vi "Periodic Tasks.vi"(8 "error in":errorcluster) -> ()   [LabVIEW 2017]
doc: "This VI runs in parallel to other tasks. It can contain as many user-defined periodic loops as you need. These can carry out PID or other sorts of timed response."
uses:
  <vilib>/Rock Robotics/WPI/Solenoid/WPI_SolenoidChannel.ctl
  Public/Documents/Cross The Road Electronics/Phoenix-LabVIEW/Motor Controller/Controls/CTRE_Phoenix_MotorControl_ControlMode.ctl
  <vilib>/Rock Robotics/WPI/Utilities/WPI_GetSetVariantRefNum.vi
  Robot Global Data.vi
  <vilib>/Rock Robotics/WPI/ThirdParty/Phoenix-LabVIEW/Motor Controller/Get/CTRE_Phoenix_MotorController_GetSelectedSensorData.vi
  <vilib>/Rock Robotics/Network Tables/NT Read String.vi
  <vilib>/Rock Robotics/WPI/Solenoid/WPI_SolenoidOpenSingle.vi
  <vilib>/Rock Robotics/WPI/Solenoid/WPI_SolenoidSetEnum.vi
  <vilib>/Rock Robotics/Network Tables/NT Read Number.vi
panel:
  out "Velocity (Raw Sensor Units per 100 ms)":i32(graph)
  in  "Min Turret":dbl
  in  "Max Turret":dbl
  in  "Min Arm":dbl
  in  "Max Arm":dbl
  in  "Min Pivot":dbl
  in  "Max Pivot":dbl
  in  "Pivot Magic?":bool=TRUE
  in  "Set Pivot Constants":bool
  in  "Pivot Constants":T1
  out "Arm Extension":i32
  out "Pivot Position":i32
  out "Turret Position":i32
  in  "Retract Solenoid Channel":T2
  out "Compressor Monitoring":bool
  out "Compressor Running":bool
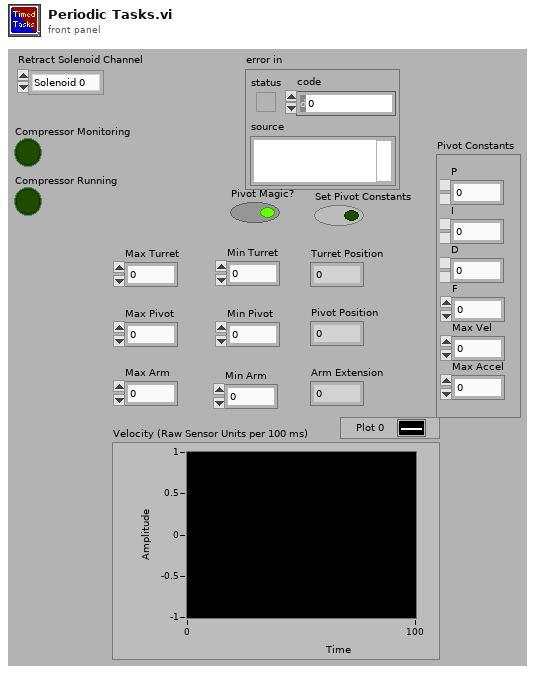
[diagram p1: front panel]
types:
  T1 = cluster{"P":dbl, "I":dbl, "D":dbl, "F":dbl, "Max Vel":dbl, "Max Accel":dbl}
  T2 = typedef "WPI_SolenoidChannel.ctl" = enum8{"Solenoid 0", "Solenoid 1", "Solenoid 2", "Solenoid 3", "Solenoid 4", "Solenoid 5", "Solenoid 6", "Solenoid 7", "Invalid"}
  T3 = typedef "WPI_CompressorDevRef.ctl" = cluster{"DevStatus":errorcluster, "Pneumatics Control Module":u8}
  T4 = typedef "WPI_SolenoidDevRef.ctl" = cluster{"DevStatus":errorcluster, "Pneumatics Control Module":u8, "Forward Solenoid Channel":T2, "Reverse Solenoid Channel":T2}
  T5 = typedef "WPI_MotorControlDeviceRef.ctl" = cluster{"DeviceStatus":errorcluster, "Type":T6, "PWM":cluster{"PWM Channel":T7, "DeadBand":T8}, "CAN":cluster{"Device Number":u8, "SetOutput VI Ref":variant, "GetOutput VI Ref":variant, "Enable VI Ref":variant, "Disable VI Ref":variant, "Data":variant}, "Invert":bool, "DIO PWM":cluster{"PWM \"Enable\" Channel":T7, "DIOChannel":T9, "PWM Rate":dbl}}
  T6 = typedef "WPI_MotorControlType.ctl" = enum16{"PWM", "CAN", "DIO PWM"}
  T7 = typedef "FPGA_DIOPWMChannel.ctl" = enum8{"PWM 0", "PWM 1", "PWM 2", "PWM 3", "PWM 4", "PWM 5", "PWM 6", "PWM 7", "PWM 8", "PWM 9", "PWM MXP 0", "PWM MXP 1", "PWM MXP 2", "PWM MXP 3", "PWM MXP 4", "PWM MXP 5", "PWM MXP 6", "PWM MXP 7", "PWM MXP 8", "PWM MXP 9", "Invalid"}
  T8 = typedef "WPI_PWMDeadband.ctl" = cluster{"Name":string, "maxPositivePwm":i32, "minPositivePwm":i32, "centerPwm":i32, "maxNegativePwm":i32, "minNegativePwm":i32, "angularRange":u16}
  T9 = typedef "FPGA_DIOChannel.ctl" = enum8{"DIO 0", "DIO 1", "DIO 2", "DIO 3", "DIO 4", "DIO 5", "DIO 6", "DIO 7", "DIO 8", "DIO 9", "DIO MXP 0", "DIO MXP 1", "DIO MXP 2", "DIO MXP 3", "DIO MXP 4", "DIO MXP 5", "DIO MXP 6", "DIO MXP 7", "DIO MXP 8", "DIO MXP 9", "DIO MXP 10", "DIO MXP 11", "DIO MXP 12", "DIO MXP 13", "DIO MXP 14", "DIO MXP 15", "SPI Port CS1", "SPI Port CS2", "SPI Port CS3", "SPI Port MISO", "SPI Port MOSI", "Invalid"}
  T10 = typedef "CTRE_Phoenix_MotorControl_ControlMode.ctl" = u16
  T11 = typedef "WPI_JoystickDevRef.ctl" = cluster{"Device":T12}
  T12 = typedef "WPI_JoystickDeviceEnum.ctl" = enum16{"USB 0", "USB 1", "USB 2", "USB 3", "USB 4", "USB 5"}
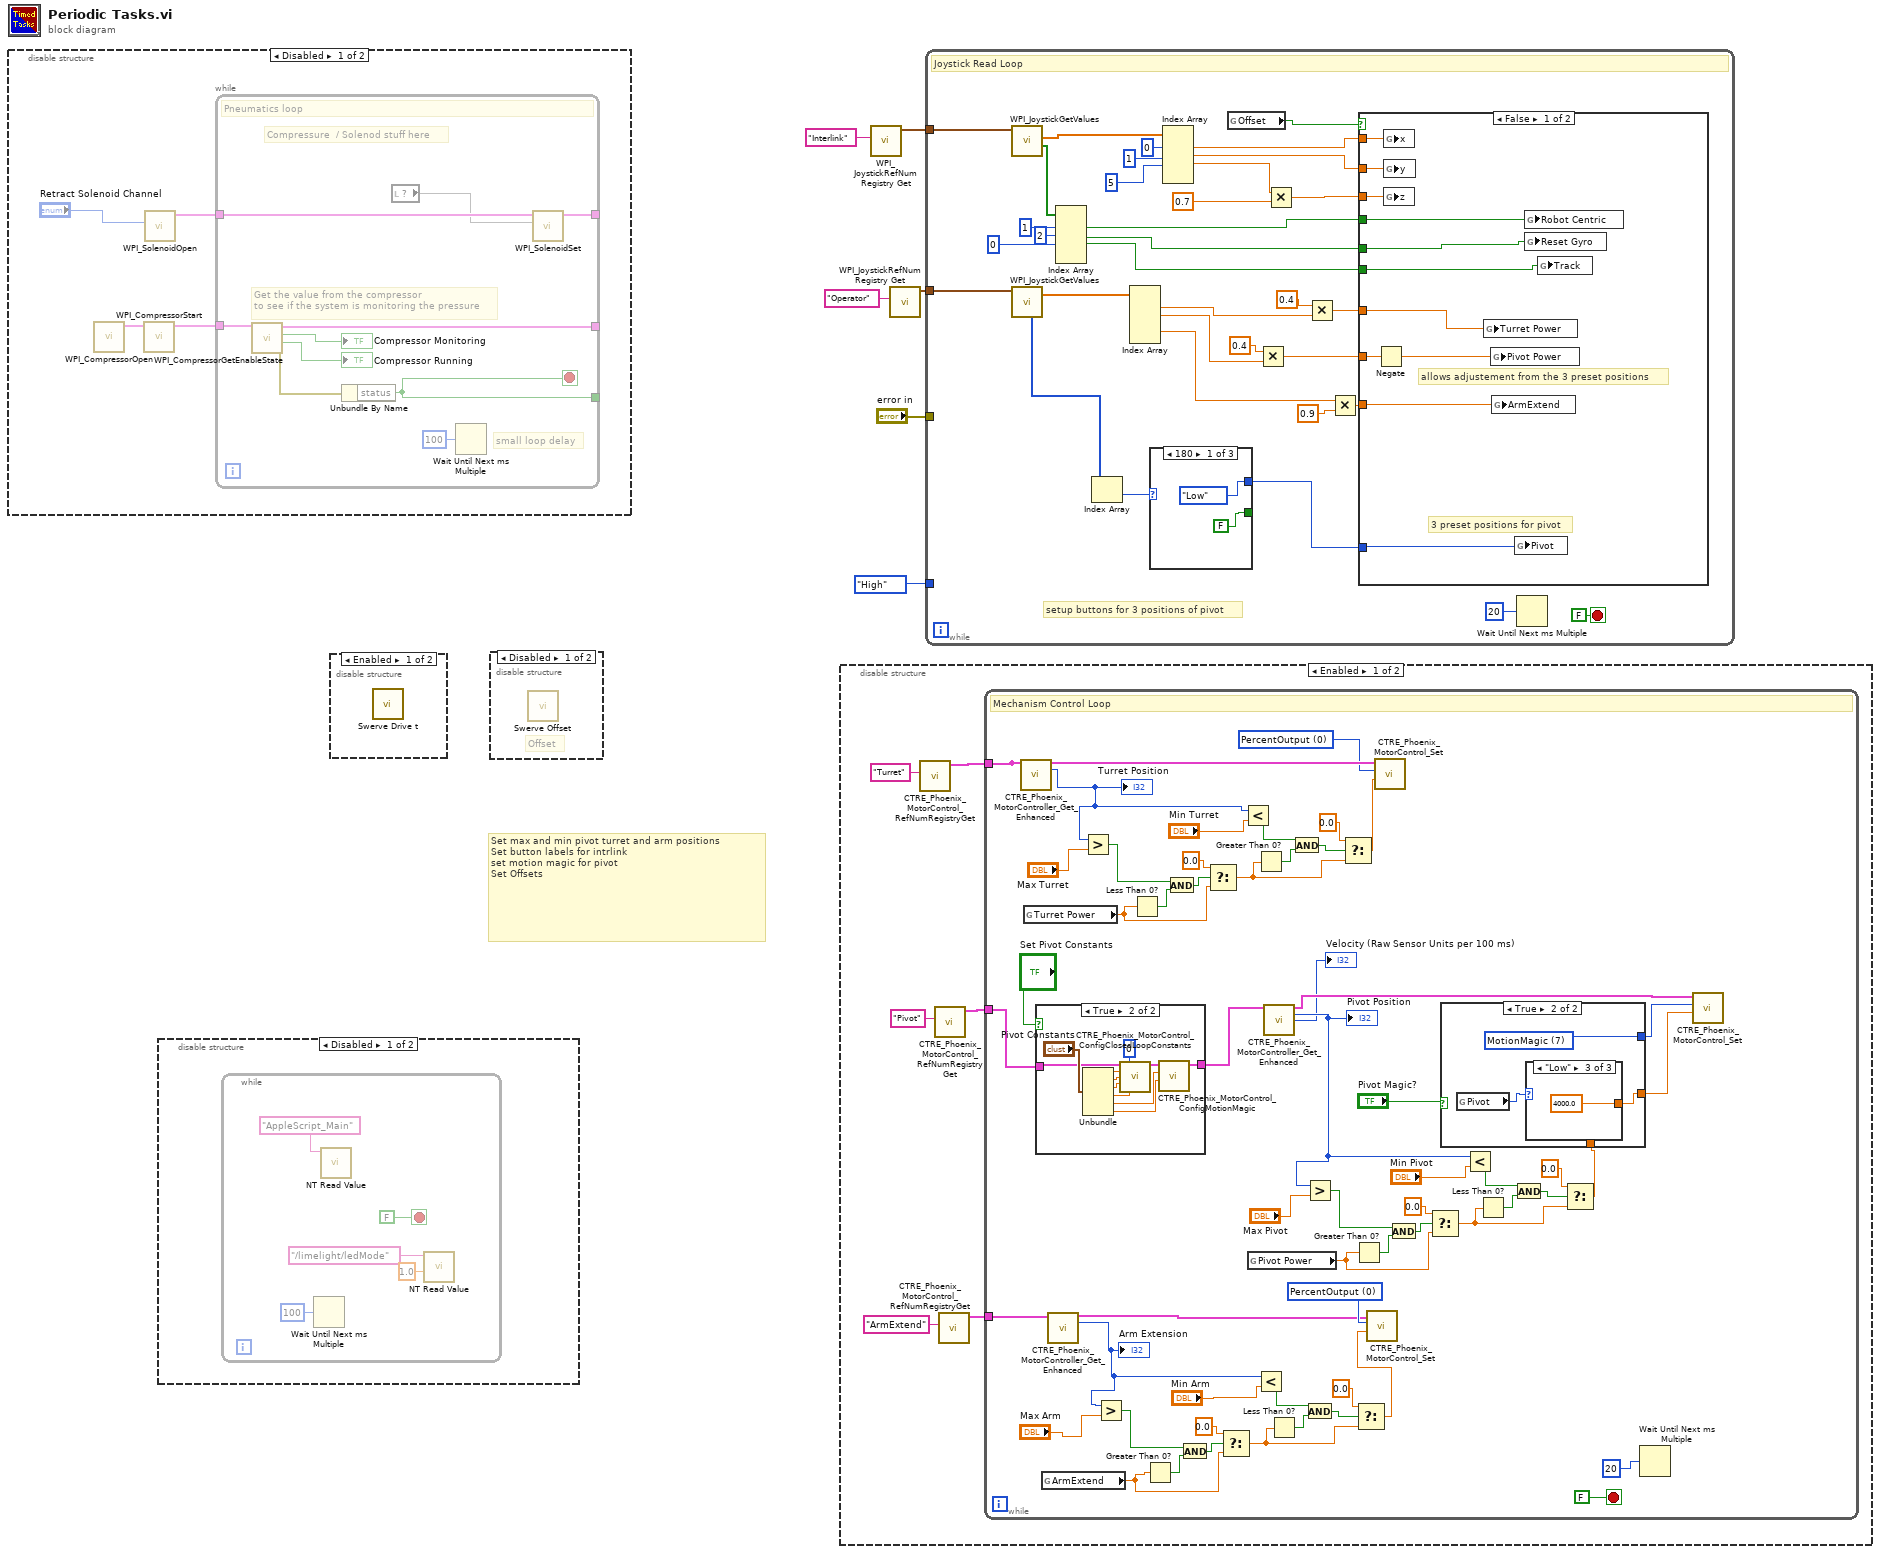
[diagram p0: block diagram]
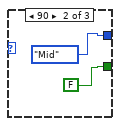
[diagram p4: hidden frame]
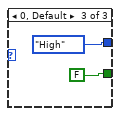
[diagram p5: hidden frame]
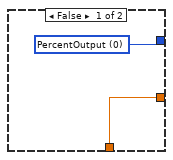
[diagram p8: hidden frame]
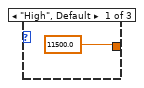
[diagram p9: hidden frame]
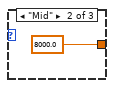
[diagram p10: hidden frame]
diagram:
  # "Set max and min pivot turret and arm positions\nSet button labels for intrlink\nset motion magic for pivot\nSet Offsets"
  n1 = disable-structure shown="Disabled" {
    frame Disabled {
      n2 = call <vilib>:"WPI_CompressorOpen.vi"() -> ("CompressorDevRef"=w7:T3)  [unwired: 14 in, 1 out]
      n3 = call <vilib>:"WPI_CompressorStart.vi"("CompressorDevRef"=w7) -> ("CompressorDevRef"=w10:T3)  [unwired: 1 in, 9 out]
      n4 = call-poly <vilib>:"WPI_SolenoidOpen.vi"("Solenoid Channel"="Retract Solenoid Channel") -> ("SolenoidDevRef"=w9:T4)  [unwired: 3 in, 7 out]
      n5 = while {
        tunnel: w10 -> [w20]
        tunnel: [w19] -> _
        tunnel: [w15] -> _
        tunnel: w9 -> [w14]
        tunnel: [w12] -> _
        stop <- w15 stop-if-true
        # "Compressure  / Solenod stuff here"
        # "small loop delay"
        # "Get the value from the compressor \nto see if the system is monitoring the pressure"
        # "Pneumatics loop"
        n6 = call <vilib>:"WPI_CompressorGetEnableState.vi"("CompressorDevRef"=w20) -> ("error out"=w16:errorcluster, "Compressor Running"=→"Compressor Running":bool, "Enabled"=→"Compressor Monitoring":bool, "CompressorDevRef"=w19:T3)  [unwired: 1 in, 6 out]
        n7 = Unbundle By Name(w16) -> ("status"=w15:bool)
        n8 = local read item#-1() -> (w11)
        n9 = Wait Until Next ms Multiple(millisecond multiple=u32 100 ("milliseconds to wait")) -> ()  [unwired: 1 out]
        n10 = call-poly <vilib>:"WPI_SolenoidSet.vi"("Value"=w11, "SolenoidDevRef"=w14) -> ("SolenoidDevRef"=w12:T4)  [unwired: 1 in, 8 out]
      }
    }
    frame Enabled {
    }
  }
  n11 = disable-structure shown="Disabled" {
    frame Disabled {
      n12 = while {
        stop <- FALSE stop-if-true
        n13 = Wait Until Next ms Multiple(millisecond multiple=u32 100) -> ()  [unwired: 1 out]
        n14 = call-poly <vilib>:"NT Read Value.vi"("Name"="AppleScript_Main") -> ()  [unwired: 9 in, 2 out]
        n15 = call-poly <vilib>:"NT Read Value.vi"("Default Value"=1.0, "Name"="/limelight/ledMode") -> ()  [unwired: 8 in, 2 out]
      }
    }
    frame Enabled {
    }
  }
  n16 = disable-structure shown="Enabled" {
    frame Enabled {
      n17 = call "Swerve Drive t.vi"() -> ()  [unwired: 16 in]
    }
    frame Disabled {
    }
  }
  n18 = disable-structure shown="Disabled" {
    frame Disabled {
      # "Offset"
      n19 = call "Swerve Offset.vi"() -> ()  [unwired: 12 in]
    }
    frame Enabled {
    }
  }
  n20 = disable-structure shown="Enabled" {
    frame Enabled {
      n21 = call <vilib>:"CTRE_Phoenix_MotorControl_RefNumRegistryGet.vi"("refnum name"="Turret") -> ("PhoenixMotorControlDevRef"=w30:T5)  [unwired: 9 in, 1 out]
      n22 = call <vilib>:"CTRE_Phoenix_MotorControl_RefNumRegistryGet.vi"("refnum name"="Pivot") -> ("PhoenixMotorControlDevRef"=w26:T5)  [unwired: 9 in, 1 out]
      n23 = call <vilib>:"CTRE_Phoenix_MotorControl_RefNumRegistryGet.vi"("refnum name"="ArmExtend") -> ("PhoenixMotorControlDevRef"=w28:T5)  [unwired: 9 in, 1 out]
      n24 = while {
        tunnel: w30 -> [w85]
        tunnel: w28 -> [w83]
        tunnel: [w85] -> _
        tunnel: w26 -> [w80]
        stop <- FALSE stop-if-true
        w84 = T10 0 items=["PercentOutput"=0, "Position"=1, "Velocity"=2, "Current"=3, "Follower"=5, "MotionProfile"=6, "MotionMagic"=7, "MotionMagicArc"=8, "MotionProfileArc"=10, "Disabled"=15] ("Control Mode")
        w86 = T10 0 items=["PercentOutput"=0, "Position"=1, "Velocity"=2, "Current"=3, "Follower"=5, "MotionProfile"=6, "MotionMagic"=7, "MotionMagicArc"=8, "MotionProfileArc"=10, "Disabled"=15] ("Control Mode")
        # "Mechanism Control Loop"
        n25 = call-poly <vilib>:"CTRE_Phoenix_MotorController_Get_Enhanced.vi"("PhoenixMotorControlDevRef"=w85) -> ("PhoenixMotorControlDevRef"=w87:T5, "Position (Raw Sensor Units)"=w34:i32)  [unwired: 11 in, 2 out]
        "Turret Position" <- w34
        n26 = global read "Robot Global Data.vi" "Turret Power"() -> (w39:dbl)
        n27 = case shown="True" "Set Pivot Constants" {
          tunnel: [w98 w100] -> w79
          tunnel: w80 -> [w98 w99]
          frame False {
          }
          frame True {
            n28 = Unbundle("Pivot Constants") -> ("P"=w103:dbl, "I"=w104:dbl, "D"=w105:dbl, "F"=w106:dbl, "Max Vel"=w107:dbl, "Max Accel"=w101:dbl)
            n29 = call <vilib>:"CTRE_Phoenix_MotorControl_ConfigClosedLoopConstants.vi"("PhoenixMotorControlDevRef"=w99, "slotIdx"=0, "P"=w103, "I"=w104, "D"=w105, "F"=w106) -> ("PhoenixMotorControlDevRef"=w102:T5)  [unwired: 8 in, 1 out]
            n30 = call <vilib>:"CTRE_Phoenix_MotorControl_ConfigMotionMagic.vi"("Acceleration"=w101, "Cruise Velocity"=w107, "PhoenixMotorControlDevRef"=w102) -> ("PhoenixMotorControlDevRef"=w100:T5)  [unwired: 7 in, 1 out]
          }
        }
        n31 = global read "Robot Global Data.vi" "ArmExtend"() -> (w49:dbl)
        n32 = call-poly <vilib>:"CTRE_Phoenix_MotorController_Get_Enhanced.vi"("PhoenixMotorControlDevRef"=w83) -> ("PhoenixMotorControlDevRef"=w82:T5, "Position (Raw Sensor Units)"=w50:i32)  [unwired: 11 in, 2 out]
        "Arm Extension" <- w50
        n33 = Greater?(x=w34, y="Max Turret") -> (0:w41:bool)
        n34 = Greater?(x=w50, y="Max Arm") -> (0:w58:bool)
        n35 = Less Than 0?(x=w39) -> (x < 0?=w42:bool)
        n36 = Greater Than 0?(x=w49) -> (x > 0?=w59:bool)
        n37 = And(x=w41, y=w42) -> (x .and. y?=w40:bool)
        n38 = And(x=w58, y=w59) -> (x .and. y?=w57:bool)
        n39 = Select(t=0.0, s=w40, f=w39) -> (s? t:f=w36:dbl)
        n40 = Select(t=0.0, s=w57, f=w49) -> (s? t:f=w51:dbl)
        n41 = Less?(x=w34, y="Min Turret") -> (x < y?=w38:bool)
        n42 = global read "Robot Global Data.vi" "Pivot Power"() -> (w62:dbl)
        n43 = Greater Than 0?(x=w36) -> (x > 0?=w37:bool)
        n44 = Less?(x=w50, y="Min Arm") -> (x < y?=w56:bool)
        n45 = call-poly <vilib>:"CTRE_Phoenix_MotorController_Get_Enhanced.vi"("PhoenixMotorControlDevRef"=w79) -> ("PhoenixMotorControlDevRef"=w77:T5, "Position (Raw Sensor Units)"=w47:i32, "Velocity (Raw Sensor Units per 100 ms)"=→"Velocity (Raw Sensor Units per 100 ms)":i32)  [unwired: 11 in, 1 out]
        "Pivot Position" <- w47
        n46 = Less Than 0?(x=w51) -> (x < 0?=w55:bool)
        n47 = And(x=w38, y=w37) -> (x .and. y?=w35:bool)
        n48 = Greater?(x=w47, y="Max Pivot") -> (0:w69:bool)
        n49 = And(x=w56, y=w55) -> (x .and. y?=w54:bool)
        n50 = Select(t=0.0, s=w35, f=w36) -> (s? t:f=w33:dbl)
        n51 = Greater Than 0?(x=w62) -> (x > 0?=w70:bool)
        n52 = Select(t=0.0, s=w54, f=w51) -> (s? t:f=w48:dbl)
        n53 = call <vilib>:"CTRE_Phoenix_MotorControl_Set.vi"("Output"=w48, "Control Mode"=w86, "PhoenixMotorControlDevRef"=w82) -> ()  [unwired: 7 in, 2 out]
        n54 = call <vilib>:"CTRE_Phoenix_MotorControl_Set.vi"("Output"=w33, "Control Mode"=w84, "PhoenixMotorControlDevRef"=w87) -> ()  [unwired: 7 in, 2 out]
        n55 = And(x=w69, y=w70) -> (x .and. y?=w68:bool)
        n56 = Select(t=0.0, s=w68, f=w62) -> (s? t:f=w65:dbl)
        n57 = Less?(x=w47, y="Min Pivot") -> (x < y?=w67:bool)
        n58 = Less Than 0?(x=w65) -> (x < 0?=w66:bool)
        n59 = And(x=w67, y=w66) -> (x .and. y?=w64:bool)
        n60 = Select(t=0.0, s=w64, f=w65) -> (s? t:f=w63:dbl)
        n61 = case shown="True" "Pivot Magic?" {
          tunnel: w63 -> [w91 _]
          tunnel: [w90 w94] -> w76
          tunnel: [w91 w92] -> w75
          frame False {
            w90 = T10 0 items=["PercentOutput"=0, "Position"=1, "Velocity"=2, "Current"=3, "Follower"=5, "MotionProfile"=6, "MotionMagic"=7, "MotionMagicArc"=8, "MotionProfileArc"=10, "Disabled"=15] ("Control Mode")
          }
          frame True {
            w94 = T10 7 items=["PercentOutput"=0, "Position"=1, "Velocity"=2, "Current"=3, "Follower"=5, "MotionProfile"=6, "MotionMagic"=7, "MotionMagicArc"=8, "MotionProfileArc"=10, "Disabled"=15] ("Control Mode")
            n62 = global read "Robot Global Data.vi" "Pivot"() -> (w93:enum16{"High", "Mid", "Low"})
            n63 = case shown="\"Low\"" w93 {
              tunnel: [11500.0 8000.0 4000.0] -> w92
              frame "High", Default {
              }
              frame "Mid" {
              }
              frame "Low" {
              }
            }
          }
        }
        n64 = Wait Until Next ms Multiple(millisecond multiple=u32 20) -> ()  [unwired: 1 out]
        n65 = call <vilib>:"CTRE_Phoenix_MotorControl_Set.vi"("Output"=w75, "Control Mode"=w76, "PhoenixMotorControlDevRef"=w77) -> ()  [unwired: 7 in, 2 out]
      }
    }
    frame Disabled {
    }
  }
  n66 = call <vilib>:"WPI_JoystickRefNum Registry Get.vi"("refnum name"="Interlink") -> ("JoystickDevRef"=w6:T11)  [unwired: 9 in, 1 out]
  n67 = call <vilib>:"WPI_JoystickRefNum Registry Get.vi"("refnum name"="Operator") -> ("JoystickDevRef"=w3:T11)  [unwired: 9 in, 1 out]
  n68 = while {
    tunnel: w6 -> [w141]
    tunnel: w3 -> [w136]
    tunnel: "error in" -> [_]
    tunnel: enum16{"High", "Mid", "Low"}."High" ("Pivot") -> [_]
    stop <- FALSE stop-if-true
    # "setup buttons for 3 positions of pivot"
    # "Joystick Read Loop"
    n69 = call <vilib>:"WPI_JoystickGetValues.vi"("JoystickDevRef"=w141) -> ("Buttons"=w129:bool[], "Axes"=w130:dbl[])  [unwired: 6 in, 3 out]
    n70 = call <vilib>:"WPI_JoystickGetValues.vi"("JoystickDevRef"=w136) -> ("Axes"=w135:dbl[], "POVs"=w114:i16[])  [unwired: 6 in, 3 out]
    n71 = Index Array(array=w129, index #1=1 ("index"), index #2=2 ("index"), index #3=0 ("index")) -> (element #1=w127:bool, element #2=w126:bool, element #3=w125:bool)  [unwired: 2 in, 2 out]
    n72 = Index Array(array=w114) -> (element=w113:i16)  [unwired: 1 in]
    n73 = Index Array(array=w135) -> (element #1=w134:dbl, element #2=w115:dbl, element #4=w110:dbl)  [unwired: 5 in, 2 out]
    n74 = case shown="180" w113 {
      tunnel: [FALSE FALSE FALSE] -> _
      tunnel: [enum16{"High", "Mid", "Low"}."Low" ("Pivot") enum16{"High", "Mid", "Low"}."Mid" ("Pivot") enum16{"High", "Mid", "Low"}."High" ("Pivot")] -> w117
      frame 180 {
      }
      frame 90 {
      }
      frame 0, Default {
      }
    }
    n75 = Index Array(array=w130, index #1=0 ("index"), index #2=1 ("index"), index #3=5 ("index")) -> (element #1=w139:dbl, element #2=w138:dbl, element #3=w123:dbl)  [unwired: 2 in, 2 out]
    n76 = global read "Robot Global Data.vi" "Offset"() -> (w140:bool)
    n77 = Multiply(x=0.4, y=w115) -> (x*y=w116:dbl)
    n78 = Multiply(x=w123, y=0.7) -> (x*y=w137:dbl)
    n79 = Multiply(x=0.4, y=w134) -> (x*y=w132:dbl)
    n80 = Multiply(x=w110, y=0.9) -> (x*y=w133:dbl)
    n81 = case shown="False" w140 {
      tunnel: w139 -> [w160 _]
      tunnel: w138 -> [w159 _]
      tunnel: w137 -> [w158 _]
      tunnel: w132 -> [w157 _]
      tunnel: w133 -> [w153 _]
      tunnel: w127 -> [w154 _]
      tunnel: w126 -> [w156 _]
      tunnel: w125 -> [w155 _]
      tunnel: w117 -> [w152 _]
      tunnel: w116 -> [w151 _]
      frame False {
        # "allows adjustement from the 3 preset positions"
        # "3 preset positions for pivot"
        n82 = Negate(x=w151) -> (-x=w150:dbl)
        n83 = global write "Robot Global Data.vi" "x"(w160) -> ()
        n84 = global write "Robot Global Data.vi" "y"(w159) -> ()
        n85 = global write "Robot Global Data.vi" "z"(w158) -> ()
        n86 = global write "Robot Global Data.vi" "Turret Power"(w157) -> ()
        n87 = global write "Robot Global Data.vi" "Pivot Power"(w150) -> ()
        n88 = global write "Robot Global Data.vi" "ArmExtend"(w153) -> ()
        n89 = global write "Robot Global Data.vi" "Pivot"(w152) -> ()
        n90 = global write "Robot Global Data.vi" "Robot Centric"(w154) -> ()
        n91 = global write "Robot Global Data.vi" "Reset Gyro"(w156) -> ()
        n92 = global write "Robot Global Data.vi" "Track"(w155) -> ()
      }
      frame True {
      }
    }
    n93 = Wait Until Next ms Multiple(millisecond multiple=u32 20) -> ()  [unwired: 1 out]
  }
